vi "Named_Serial_Comms.vi"(0 "Channel Name":string, 1 "Write":string, 2 "Timeout/ms":u32=500, 4 "!Error retries":i32=10, 6 "!Timeout retries":i32=3, 9 "Port Name":refnum<visa-resource-name>, 11 "Term Grep":string="\r$", 12 "Log Errors?":bool=TRUE, 13 "Terminate Count":i32) -> (3 "Read":string="This is simulation mode", 8 "Error Description":string, 10 "millisecond timer value":u32, 14 "Timed out":bool, 15 "Serial Error":bool)   [LabVIEW 2022 SP3]
doc: "The Serial Communication VI performs bidirectional communication with a port. It initializes the port, writes a string to the port, and performs a read with timeout. The Read with Timeout will wait until a terminating character is received or the time limit is up, whichever comes first.\nThe initialisation parameters, terminating character, and timeout, are all set in the Serial Setup Global."
uses:
  subVIs/Port_Params.ctl
  <vilib>/Instr/_visa.llb/VISA Find Search Mode.ctl
  <vilib>/Instr/serial.llb/serpConfig.vi
  Anemometry/Anemometry Sub Vis/Globals/Preference_global.vi
panel:
  in  "Tab Control":T1(tab)
  in  "Uppercase?":bool
  in  "Append Return?":bool
  in  "!stop":bool
  out "Terminated?":bool
  in  "Force setup reload":bool
  in  "Save Setups?":bool
  out "Buffer Trash":string
  out "byte count":u32
  out "Port Settings Array":T2[](array[typedef]) {"flow control etc."."parity err byte" format="%.0x"; "flow control etc."."XON byte" format="%.0x"; "flow control etc."."XOFF byte" format="%.0x"; "data bits" min=5 max=8 step=1}
  out "enumerated ports":string[](array[string])
  out "Ports having file settings":string[](array[string])
  out "Port Initialised?":bool[](array[boolean])
  out "Setting Number":i32
  out "Port Initialisation Parameters":T2={"Name"="", "flow control etc."={"input XON/XOFF"=FALSE, "input HW Handshake"=FALSE, "input alt HW HShk"=FALSE, "output XON/XOFF"=FALSE, "output HW Handshake"=FALSE, "output alt HW HShk"=FALSE, "XOFF byte "=0, "XON byte"=0, "parity err byte"=0}, "buffer size"=0, "baud rate"=9600, "data bits"=8, "stop bits"=enum."1 bit", "parity"=enum."no parity"} {"flow control etc."."parity err byte" format="%.0x"; "flow control etc."."XON byte" format="%.0x"; "flow control etc."."XOFF byte" format="%.0x"; "data bits" min=5 max=8 step=1}
  out "isGillUsonic":bool
  out "etherComms":errorcluster
  out "Audit trail":string[](array[string])
  out "Case":string="Simulate"
  out "Initialise error":i32
  out "Write error":i32
  out "n-bytes error code":i32
  out "read error code":i32
  out "Close Port error":i32
  out "load setups error":bool
  out "PortType":string
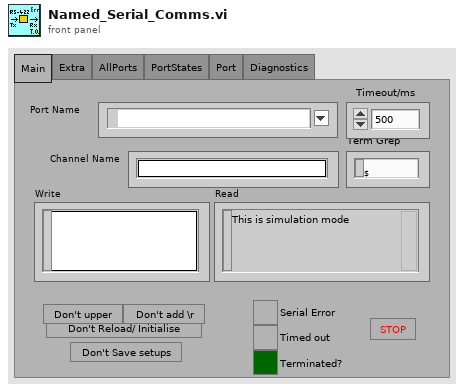
[diagram p1: front panel]
types:
  T1 = enum32{"Main", "Extra", "AllPorts", "PortStates", "Port", "Diagnostics"}
  T2 = typedef "Port_Params.ctl" = cluster{"Name":string, "flow control etc.":cluster{"input XON/XOFF":bool, "input HW Handshake":bool, "input alt HW HShk":bool, "output XON/XOFF":bool, "output HW Handshake":bool, "output alt HW HShk":bool, "XOFF byte ":u8, "XON byte":u8, "parity err byte":u16}, "buffer size":u16, "baud rate":u32, "data bits":u16, "stop bits":enum16{"1 bit", "1.5 bits", "2 bits"}, "parity":enum16{"no parity", "odd parity", "even parity", "mark parity", "space parity"}}
  T3 = typedef "VISA Find Search Mode.ctl" = u32
  T4 = cluster{"input XON/XOFF":bool, "input HW Handshake":bool, "input alt HW HShk":bool, "output XON/XOFF":bool, "output HW Handshake":bool, "output alt HW HShk":bool, "XOFF byte ":u8, "XON byte":u8, "parity err byte":u16}
  T5 = enum16{"no parity", "odd parity", "even parity", "mark parity", "space parity"}
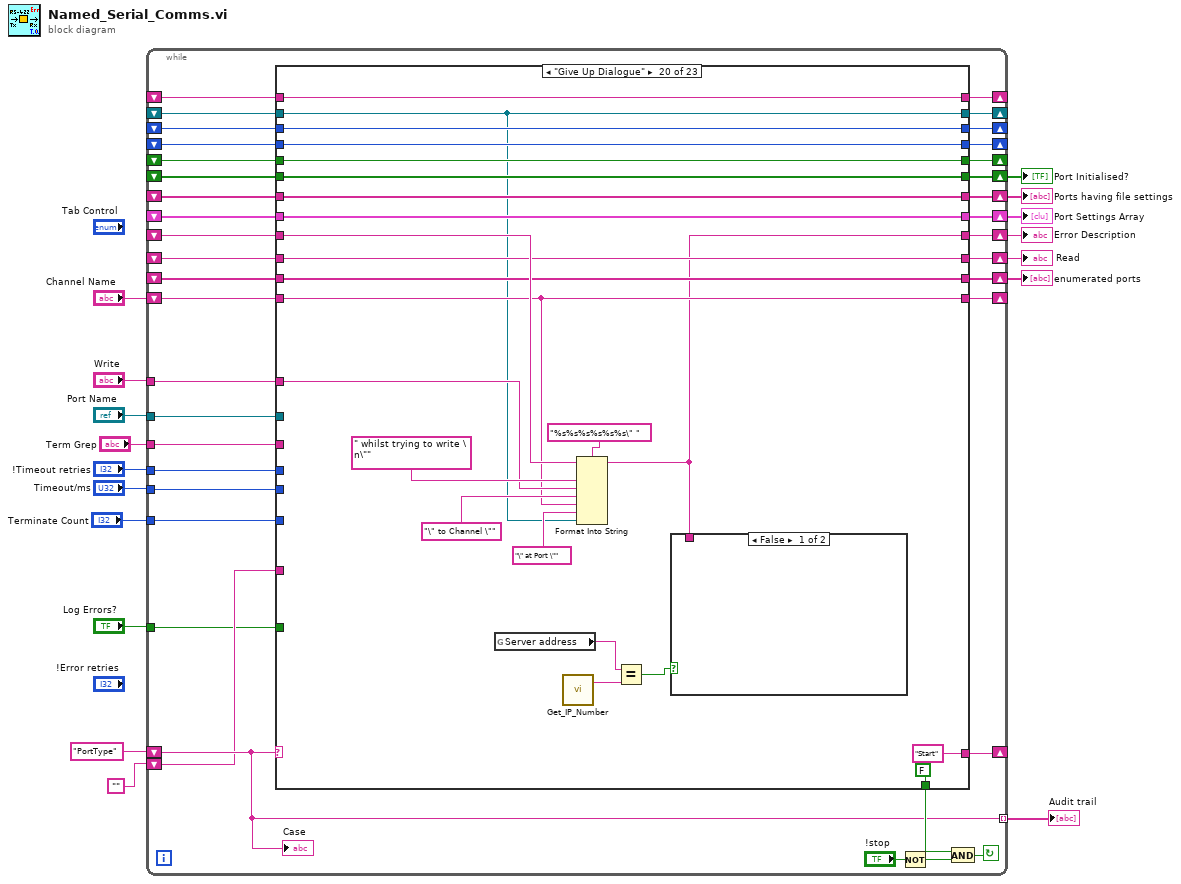
[diagram p0: block diagram]
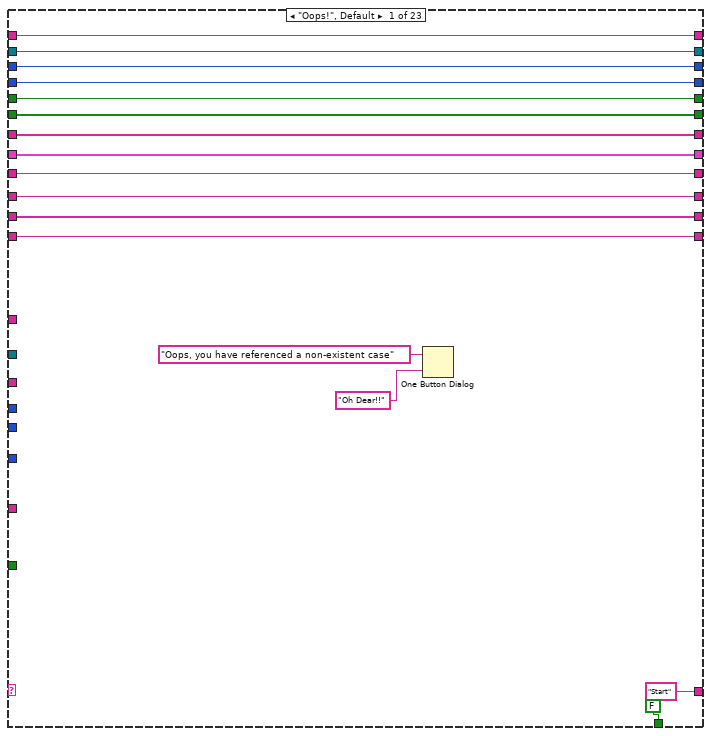
[diagram p2: hidden frame]
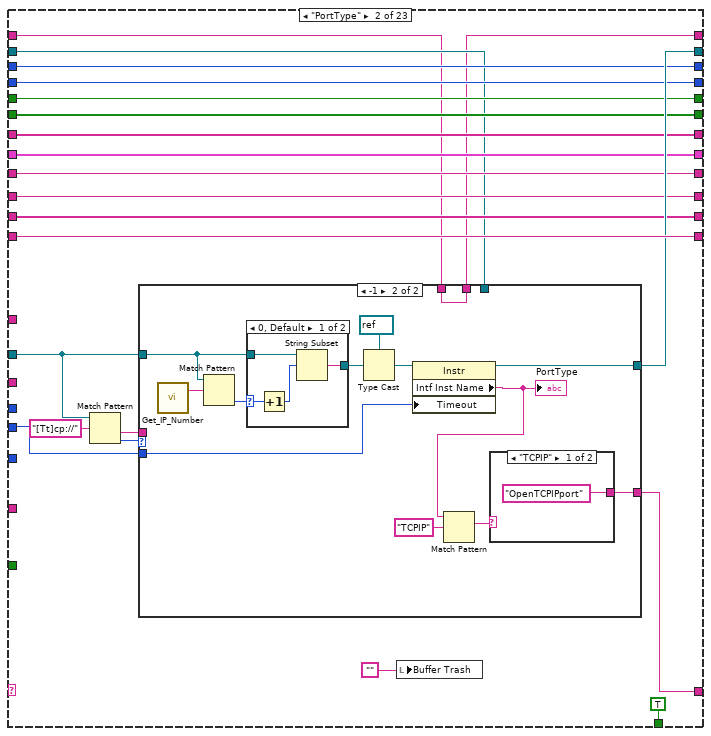
[diagram p3: hidden frame]
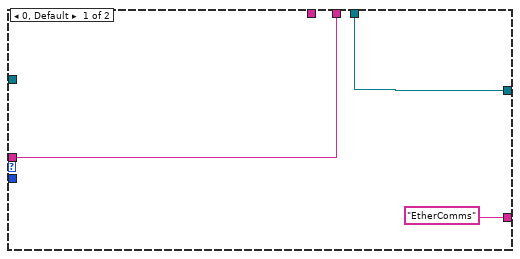
[diagram p4: hidden frame]
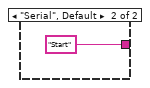
[diagram p5: hidden frame]
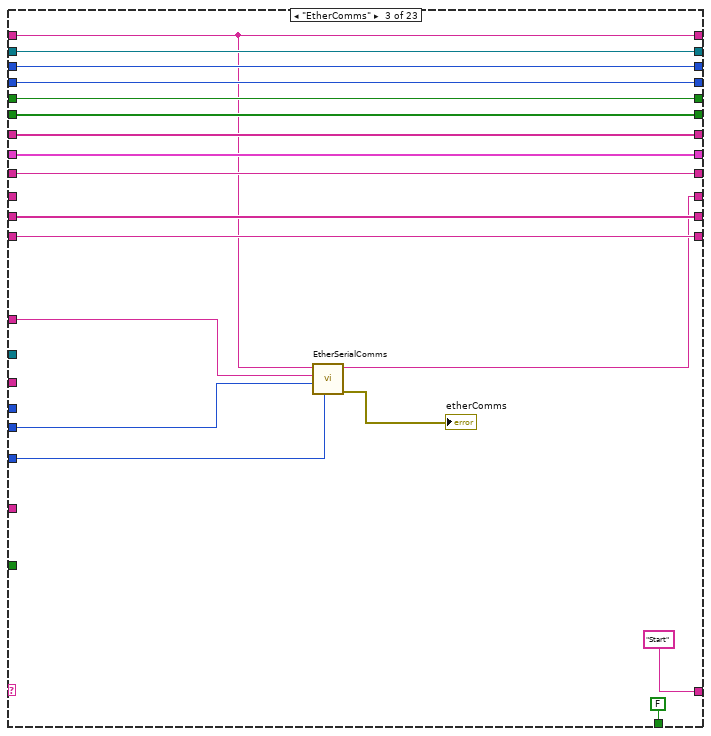
[diagram p7: hidden frame]
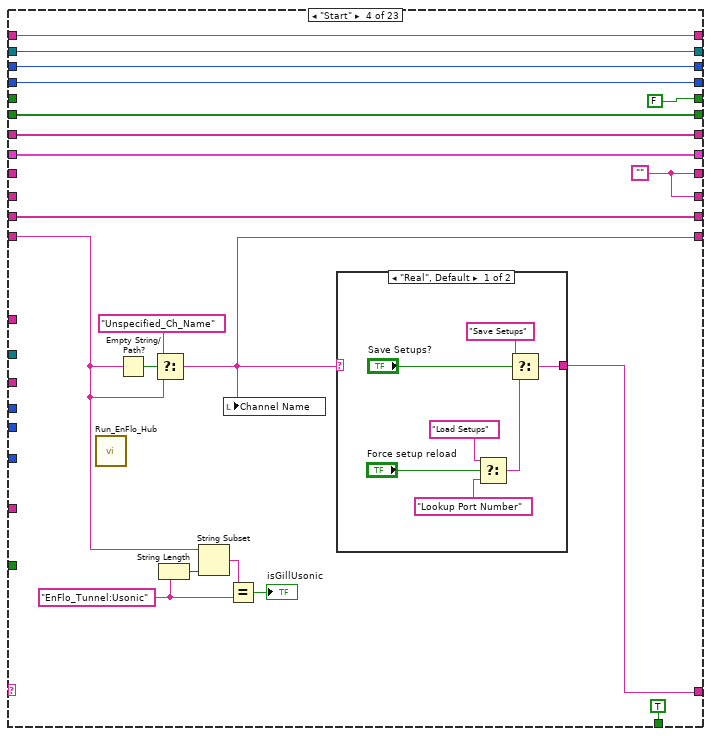
[diagram p8: hidden frame]
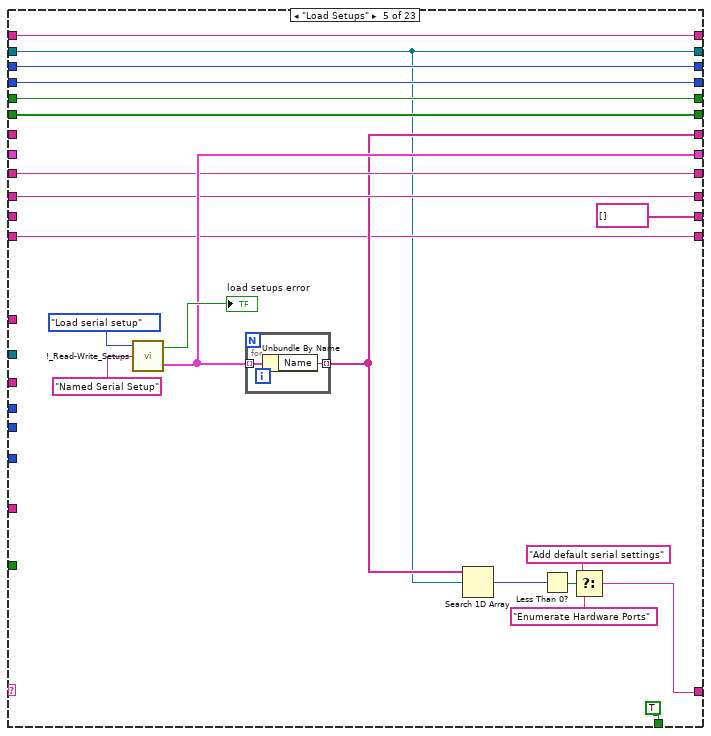
[diagram p10: hidden frame]
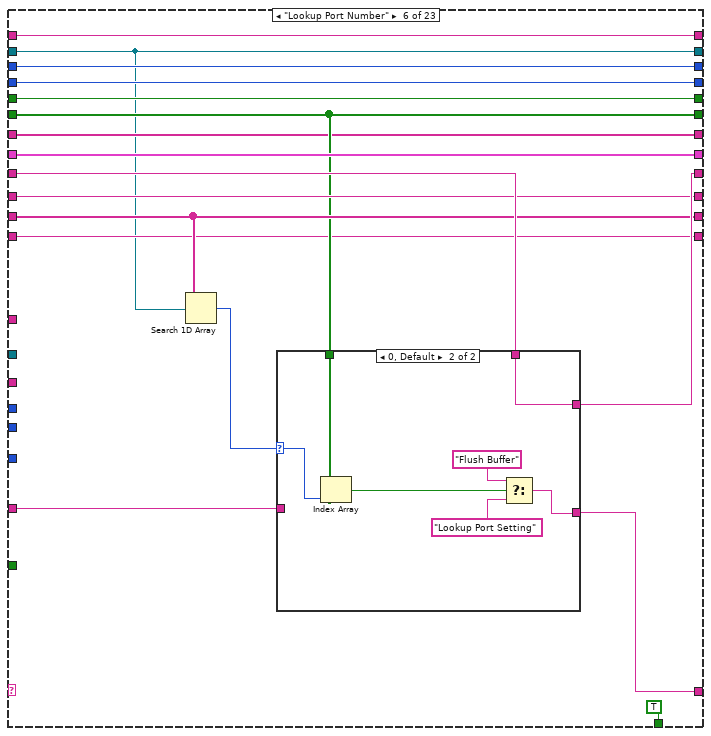
[diagram p11: hidden frame]
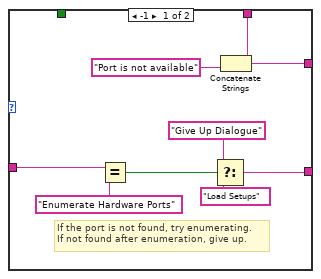
[diagram p12: hidden frame]
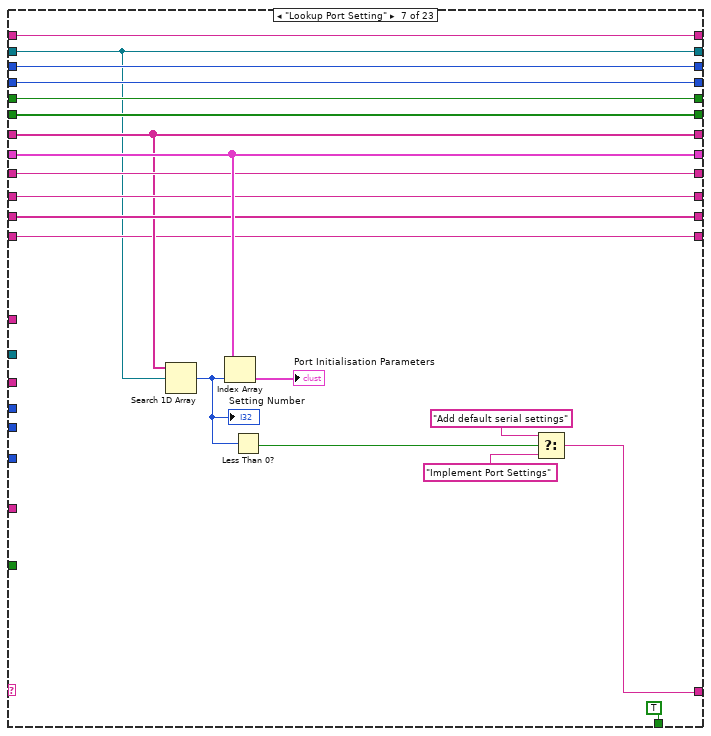
[diagram p13: hidden frame]
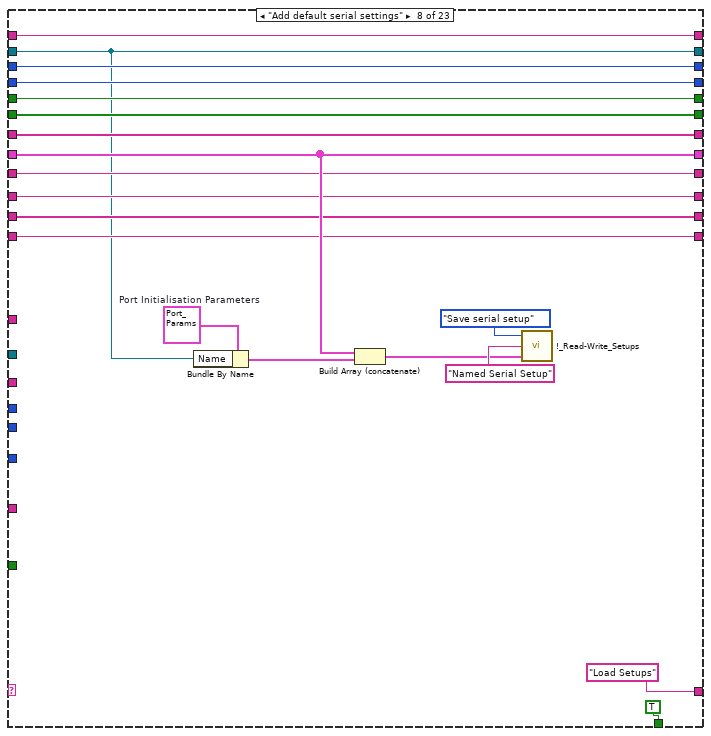
[diagram p14: hidden frame]
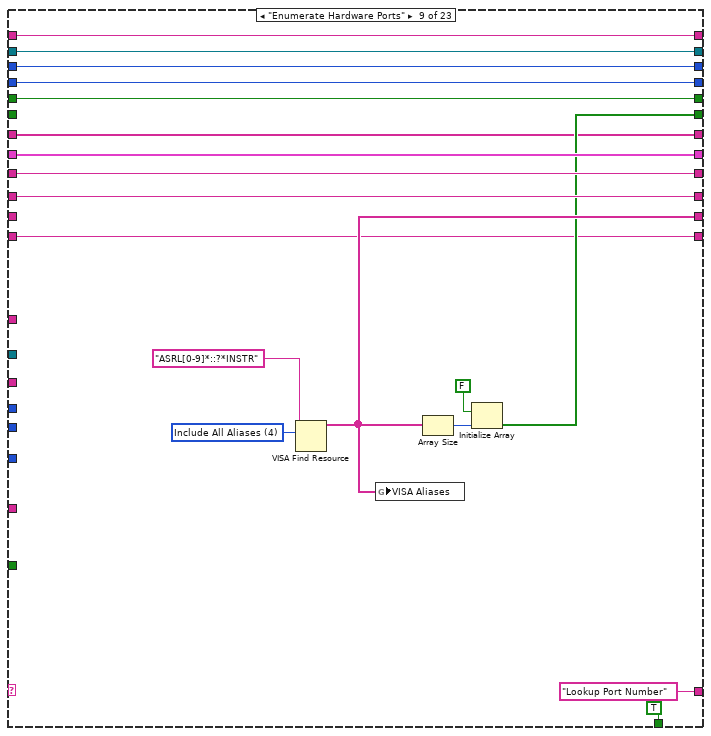
[diagram p15: hidden frame]
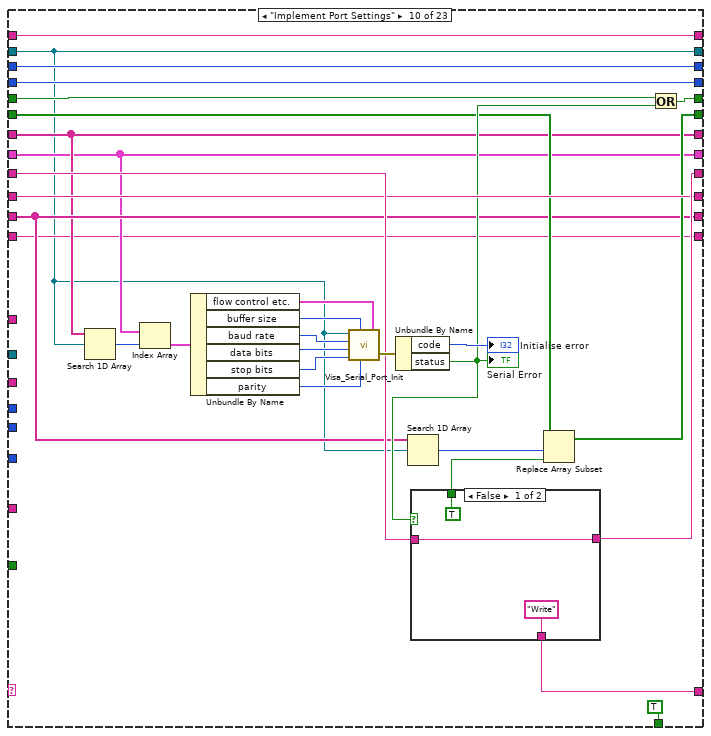
[diagram p16: hidden frame]
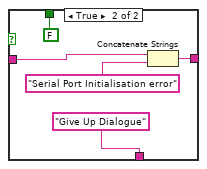
[diagram p17: hidden frame]
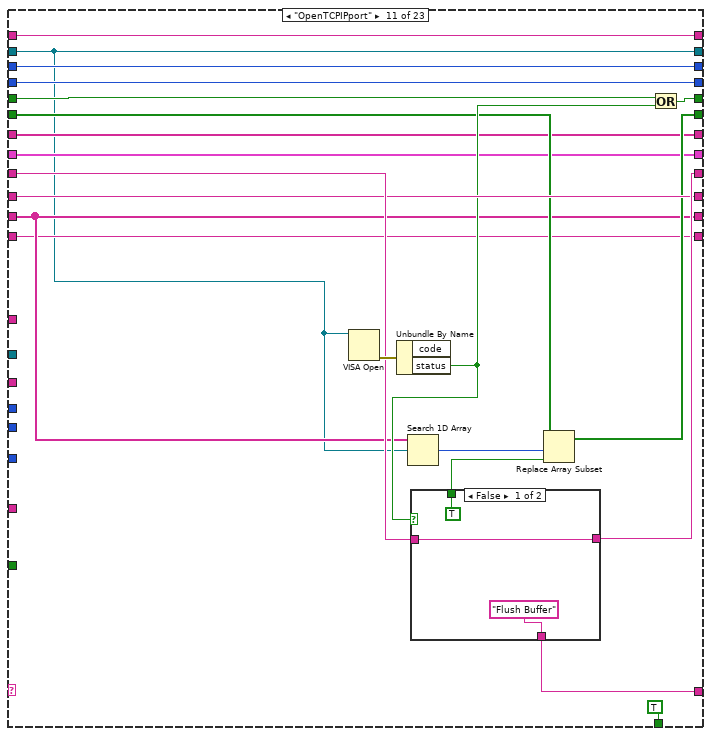
[diagram p18: hidden frame]
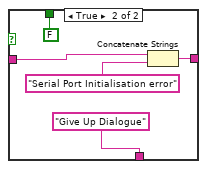
[diagram p19: hidden frame]
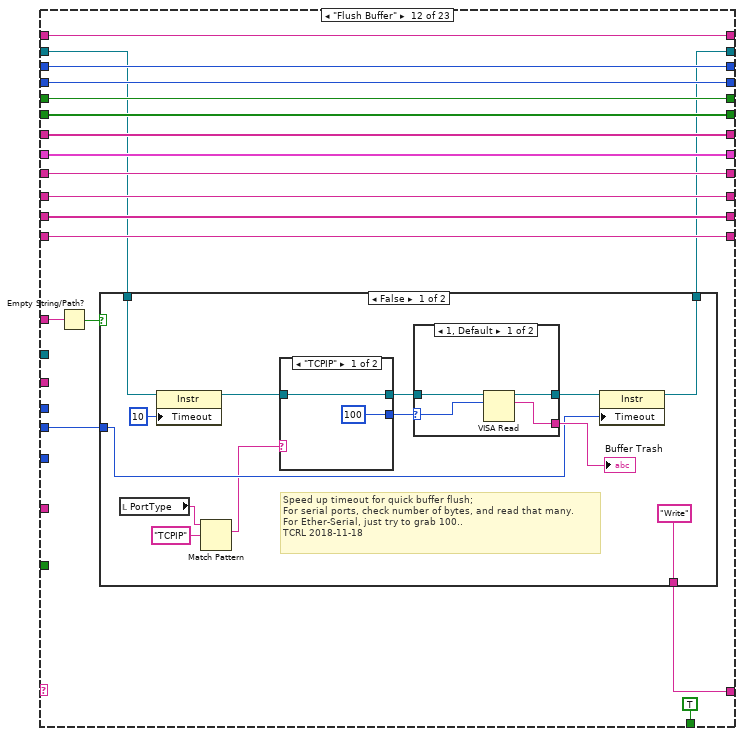
[diagram p20: hidden frame]
diagram:
  n1 = while {
    tunnel: "!Timeout retries" -> [w47]
    shift-left: "" -> [w48]
    tunnel: [w49] -> w5 mode=indexing
    shift-left: "PortType" -> [w49]
    shift-right: [w50] -> _
    tunnel: "Write" -> [w55]
    tunnel: "Log Errors?" -> [w46]
    shift-right: [w45] -> w12
    shift-left: _ -> [w44]
    shift-right: [w42] -> w11
    shift-left: _ -> [w43]
    shift-right: [w41] -> w10
    shift-left: _ -> [w40]
    shift-right: [w39] -> w9
    shift-left: _ -> [w38]
    shift-right: [w37] -> _
    shift-left: _ -> [w36]
    shift-right: [w35] -> w8
    shift-left: _ -> [w34]
    shift-right: [w32] -> w7
    shift-left: _ -> [w33]
    shift-right: [w29] -> _
    shift-left: _ -> [w28]
    shift-right: [w31] -> _
    shift-left: _ -> [w30]
    shift-right: [w26] -> _
    shift-left: "Channel Name" -> [w27]
    shift-right: [w25] -> _
    shift-left: _ -> [w24]
    tunnel: "Port Name" -> [w23]
    shift-right: [w22] -> _
    shift-left: _ -> [w21]
    tunnel: "Timeout/ms" -> [w20]
    tunnel: "Terminate Count" -> [w19]
    tunnel: "Term Grep" -> [w18]
    stop <- w53 continue-if-true
    n2 = case shown="\"Give Up Dialogue\"" w49 {
      tunnel: w55 -> [_ _ w121 _ _ _ _ _ _ _ _ w344 w405 _ _ _ _ _ w604 w631 _ _ _]
      tunnel: ["Start" ("f") w74 "Start" w154 w165 w201 w223 "Load Setups" ("f") "Lookup Port Number" w297 w332 w342 w402 "Bytes At Serial Port?" ("f") w472 w526 w552 w594 "Start" "Start" "Start" "Start" ("f") "Load Setups" ("f")] -> w50
      tunnel: [FALSE TRUE FALSE TRUE TRUE TRUE TRUE TRUE TRUE TRUE TRUE TRUE TRUE TRUE TRUE TRUE TRUE TRUE FALSE FALSE TRUE FALSE TRUE] -> w54
      tunnel: w48 -> [_ _ _ _ _ w200 _ _ _ _ _ _ _ _ _ _ _ _ _ _ _ _ _]
      tunnel: w47 -> [_ _ _ _ _ _ _ _ _ _ _ _ w400 _ w471 _ _ _ _ _ _ _ _]
      tunnel: w46 -> [_ _ _ _ _ _ _ _ _ _ _ _ _ _ _ _ _ _ w610 _ _ _ _]
      tunnel: [w67 w86 w128 w152 w179 w199 w234 w249 w270 w281 w318 w358 w399 w451 w470 w518 w547 w590 w609 w628 w650 w667 w681] -> w45
      tunnel: w44 -> [w67 w86 w128 w152 _ w199 w234 w249 w270 w281 w318 w358 w399 w451 w470 w518 w547 w590 w609 w628 w650 w667 w681]
      tunnel: w43 -> [w66 w85 w127 _ w178 w198 w233 w248 w269 w292 w328 w357 w397 w450 w469 w517 w546 w589 w608 w627 w649 w666 w680]
      tunnel: [w66 w85 w127 w151 w178 w197 w233 w248 w269 w293 w329 w357 w398 w450 w469 w517 w546 w589 w608 w616 w649 w666 w680] -> w42
      tunnel: [w65 w84 w119 w151 w177 w196 w232 w247 w268 w291 w327 w356 w396 "" w468 w516 w545 w588 w607 w626 w648 "Simulated Serial Read" w679] -> w41
      tunnel: w40 -> [w65 w84 _ _ w177 w196 w232 w247 w268 w291 w327 w356 w396 _ w468 w515 w545 w588 w607 w626 w648 _ w679]
      tunnel: [w64 w83 w126 w150 string[] [] ("enumerated ports") w195 w231 w246 w267 w283 w320 w355 w395 w448 w467 w514 w544 w587 w606 w625 w647 w664 w678] -> w39
      tunnel: w38 -> [w64 w83 w126 w150 _ w195 w231 w246 _ w283 w320 w355 w395 w448 w467 w514 w544 w587 w606 w625 w647 w664 w678]
      tunnel: [w63 w89 w131 FALSE w175 w194 w230 w245 w266 w289 w325 w354 w394 w447 w466 w513 w543 w585 w605 w624 w646 w663 w677] -> w37
      tunnel: w36 -> [w63 w89 w131 _ w175 w194 w230 w245 w266 w290 w326 w354 w394 w447 w466 w513 w543 w586 w605 w624 w646 w663 w677]
      tunnel: [w62 w88 w130 w148 w174 w192 w229 w244 w265 w286 w322 w353 w393 w446 w465 w512 w542 w583 w603 w623 w645 w662 w676] -> w35
      tunnel: w34 -> [w62 w88 w130 w148 w174 w192 w229 w244 _ w285 w321 w353 w393 w446 w465 w512 w542 w583 w603 w623 w645 w662 w676]
      tunnel: [w61 w87 w129 w147 w173 w191 w228 w243 w264 w282 w319 w352 w392 w445 w464 w511 w541 w582 w602 w622 w644 w661 w675] -> w32
      tunnel: w33 -> [w61 w87 w129 w147 _ w191 w228 w243 w264 w282 w319 w352 w392 w445 w464 w511 w541 w582 w602 w622 w644 w661 w675]
      tunnel: [w60 w91 w133 w146 w172 w190 w227 w242 w263 w279 w317 w351 w391 w444 w462 w507 w540 w581 w601 w621 w643 w660 w674] -> w31
      tunnel: w30 -> [w60 w91 w133 w146 w172 w190 w227 w242 w263 w279 w317 w351 w391 _ w462 w507 w540 w581 w601 w621 w643 w660 w674]
      tunnel: [w59 w90 w132 w145 w171 w189 w226 w241 w262 w278 w316 w350 w390 w443 w463 w506 w539 w580 w600 w620 w642 w659 w673] -> w29
      tunnel: w28 -> [w59 w90 w132 w145 w171 w189 w226 w241 w262 w278 w316 w350 w390 w443 _ w506 w539 w580 w600 w620 w642 w659 w673]
      tunnel: w27 -> [w58 w93 w134 w137 w170 w188 w225 w240 w260 w277 w315 w349 w388 w442 w461 w505 w538 w579 w597 w619 w641 w658 w672]
      tunnel: [w58 w93 w134 w135 w170 w188 w225 w240 w260 w277 w315 w349 w388 w442 w461 w505 w538 w579 w597 w619 w641 w658 w672] -> w26
      tunnel: [w57 w92 w123 w142 w164 w187 w221 w239 w259 w276 w313 w346 w387 w441 w459 w504 w537 w578 w599 w618 w640 w657 w671] -> w25
      tunnel: w24 -> [w57 w77 w123 w142 w164 w187 w221 w239 w259 w276 w313 w345 w387 w441 w459 w504 w537 w578 w599 w618 w640 w657 w671]
      tunnel: w23 -> [_ w81 _ _ _ _ _ _ _ _ _ _ _ _ _ _ _ _ _ _ _ _ _]
      tunnel: [w56 w76 w122 w141 w163 w186 w222 w238 w258 w275 w314 w348 w386 w440 w460 w503 w536 w577 w598 w617 w639 w656 w670] -> w22
      tunnel: w21 -> [w56 w75 w122 w141 w163 w186 w222 w238 w258 w275 w314 w348 w386 w440 w460 w503 w536 w577 w598 w617 w639 w656 w670]
      tunnel: w20 -> [_ w73 w120 _ _ _ _ _ _ _ _ w347 _ _ _ _ _ w576 _ _ _ _ _]
      tunnel: w19 -> [_ _ w117 _ _ _ _ _ _ _ _ _ _ _ w458 _ w535 _ _ _ _ _ _]
      tunnel: w18 -> [_ _ _ _ _ _ _ _ _ _ _ _ _ _ w457 _ w534 _ _ _ _ _ _]
      frame "Oops!", Default {
        n3 = One Button Dialog(message="Oops, you have referenced a non-existent case", button name ("OK")="Oh Dear!!") -> ()  [unwired: 1 out]
      }
      frame "PortType" {
        n4 = Match Pattern(string=w81, regular expression="[Tt]cp://") -> (after substring=w78:string, offset past match=w79:i32)  [unwired: 1 in, 2 out]
        n5 = case shown="-1" w79 {
          tunnel: [w96 w100] -> w92
          tunnel: w81 -> [_ w105]
          tunnel: w78 -> [w95 _]
          tunnel: w77 -> [w96 _]
          tunnel: [w95 w104] -> w76
          tunnel: w75 -> [_ w104]
          tunnel: ["EtherComms" w103] -> w74
          tunnel: w73 -> [_ w102]
          frame 0, Default {
          }
          frame -1 {
            n6 = call "Get_IP_Number.vi"() -> ("IP Number"=w108:string)  [unwired: 1 out]
            n7 = Match Pattern(string=w105, regular expression=w108) -> (offset past match=w107:i32)  [unwired: 4 out]
            n8 = case shown="0, Default" w107 {
              selector: w107 -> [w112 _]
              tunnel: [w113 w116] -> w109
              tunnel: w105 -> [w114 w116]
              frame 0, Default {
                n9 = Increment(x=w112) -> (x+1=w115:i32)
                n10 = String Subset(string=w114, offset (0)=w115) -> (substring=w113:string)  [unwired: 1 out]
              }
              frame -1 {
              }
            }
            n11 = Type Cast(type=refnum<visa-resource-name> refnum ("dup VISA resource name"), x=w109) -> (*(type *) &x=w101:refnum<visa-resource-name>)
            n12 = property class="Instr"(reference=w101, "Timeout"=w102) -> (reference out=w100:refnum<visa-resource-name>, "Intf Inst Name"=w97:string)  [unwired: 1 in, 1 out]
            "PortType" <- w97
            n13 = Match Pattern(string=w97, regular expression="TCPIP") -> (match substring=w98:string)  [unwired: 1 in, 3 out]
            n14 = case shown="\"TCPIP\"" w98 {
              tunnel: ["OpenTCPIPport" "Start"] -> w103
              frame "TCPIP" {
              }
              frame "Serial", Default {
              }
            }
          }
        }
        n15 = local write "Buffer Trash"("") -> ()
      }
      frame "EtherComms" {
        n16 = call "EtherSerialComms.vi"("byteCount"=w117, "Timeout/ms"=w120, "Write"=w121, "Port Name"=w122) -> ("error out"=→"etherComms":errorcluster, "data out"=w119:string)  [unwired: 5 in, 1 out]
      }
      frame "Start" {
        w140 = "EnFlo_Tunnel:Usonic"
        w151 = ""
        n17 = call "Run_EnFlo_Hub.vi"() -> ()  [unwired: 1 in, 7 out]
        n18 = Empty String/Path?(string/path=w137) -> (empty?=w144:bool)
        n19 = Select(t="Unspecified_Ch_Name", s=w144, f=w137) -> (s? t:f=w135:string)
        n20 = String Length(string=w140) -> (length=w138:i32)
        n21 = String Subset(string=w137, length (rest)=w138) -> (substring=w139:string)  [unwired: 1 out]
        n22 = local write "Channel Name"(w135) -> ()
        n23 = Equal?(x=w139, y=w140) -> (x = y?=→"isGillUsonic":bool)
        n24 = case shown="\"Real\", Default" w135 {
          selector: w135 -> [_ w162]
          tunnel: [w157 w162] -> w154
          frame "Real", Default {
            n25 = Select(t="Load Setups" ("f"), s="Force setup reload", f="Lookup Port Number") -> (s? t:f=w158:string)
            n26 = Select(t="Save Setups", s="Save Setups?", f=w158) -> (s? t:f=w157:string)
          }
          frame "Simulate" {
          }
        }
      }
      frame "Load Setups" {
        n27 = call "!_Read-Write_Setups.vi"("Setup Name"="Named Serial Setup", "Mode"=enum16{"Load serial setup", "Save serial setup"}."Load serial setup") -> ("Port Settings Array Out"=w179:T2[], "error unflattening"=→"load setups error":bool)  [unwired: 1 in]
        n28 = for {
          tunnel: w179 -> [w185] mode=indexing
          tunnel: [w184] -> w173 mode=indexing
          n29 = Unbundle By Name(w185) -> ("Name"=w184:string)
        }
        n30 = Search 1D Array(1D array=w173, element=w164) -> (index of element=w169:i32)  [unwired: 1 out]
        n31 = Less Than 0?(x=w169) -> (x < 0?=w168:bool)
        n32 = Select(t="Add default serial settings", s=w168, f="Enumerate Hardware Ports") -> (s? t:f=w165:string)
      }
      frame "Lookup Port Number" {
        n33 = Search 1D Array(1D array=w195, element=w187) -> (index of element=w193:i32)  [unwired: 1 out]
        n34 = case shown="0, Default" w193 {
          selector: w193 -> [_ w212]
          tunnel: [w211 w218] -> w201
          tunnel: w200 -> [w208 _]
          tunnel: w198 -> [w204 w214]
          tunnel: [w203 w214] -> w197
          tunnel: w192 -> [_ w213]
          frame -1 {
            # "If the port is not found, try enumerating.\nIf not found after enumeration, give up."
            n35 = Equal?(x=w208, y="Enumerate Hardware Ports" ("f")) -> (x = y?=w210:bool)
            n36 = Select(t="Give Up Dialogue" ("f"), s=w210, f="Load Setups") -> (s? t:f=w211:string)
            n37 = Concatenate Strings(w204, "Port is not available" ("Error Description")) -> (w203:string)
          }
          frame 0, Default {
            n38 = Index Array(array=w213, index=w212) -> (element=w217:bool)
            n39 = Select(t="Flush Buffer" ("f"), s=w217, f="Lookup Port Setting") -> (s? t:f=w218:string)
          }
        }
      }
      frame "Lookup Port Setting" {
        n40 = Search 1D Array(1D array=w228, element=w221) -> (index of element=w235:i32)  [unwired: 1 out]
        "Setting Number" <- w235
        n41 = Index Array(array=w234, index=w235) -> (element=→"Port Initialisation Parameters":T2)
        n42 = Less Than 0?(x=w235) -> (x < 0?=w224:bool)
        n43 = Select(t="Add default serial settings", s=w224, f="Implement Port Settings") -> (s? t:f=w223:string)
      }
      frame "Add default serial settings" {
        w256 = T2 {"Name"="", "flow control etc."={"input XON/XOFF"=FALSE, "input HW Handshake"=FALSE, "input alt HW HShk"=FALSE, "output XON/XOFF"=FALSE, "output HW Handshake"=FALSE, "output alt HW HShk"=FALSE, "XOFF byte "=19, "XON byte"=17, "parity err byte"=0}, "buffer size"=200, "baud rate"=9600, "data bits"=8, "stop bits"=enum."1 bit", "parity"=enum."no parity"}  # Port Initialisation Parameters
        n44 = Bundle By Name(cluster=w256, "Name"=w239) -> (w255:T2)
        n45 = Build Array (concatenate)(w249, w255) -> (w252:T2[])
        n46 = call "!_Read-Write_Setups.vi"("Port Settings Array In"=w252, "Setup Name"="Named Serial Setup", "Mode"=enum16{"Load serial setup", "Save serial setup"}."Save serial setup") -> ()  [unwired: 2 out]
      }
      frame "Enumerate Hardware Ports" {
        w261 = T3 4 items=["Canonical Names Only"=0, "Aliases Only"=2, "Include Matching Aliases"=3, "Include All Aliases"=4] ("Search Mode")
        n47 = VISA Find Resource(10:w261, 11:"ASRL[0-9]*::?*INSTR" ("expression (\"?*\")")) -> (3:w267:string[])  [unwired: 1 in, 2 out]
        n48 = global write "serpConfig.vi" "VISA Aliases"(w267) -> ()
        n49 = Array Size(array=w267) -> (size(s)=w272:i32)
        n50 = Initialize Array(FALSE, w272) -> (w265:bool[])
      }
      frame "Implement Port Settings" {
        n51 = Search 1D Array(1D array=w282, element=w276) -> (index of element=w284:i32)  [unwired: 1 out]
        n52 = Index Array(array=w281, index=w284) -> (element=w280:T2)
        n53 = Unbundle By Name(w280) -> ("flow control etc."=w304:T4, "buffer size"=w303:u16, "baud rate"=w302:u32, "data bits"=w301:u16, "stop bits"=w300:enum16{"1 bit", "1.5 bits", "2 bits"}, "parity"=w299:T5)
        n54 = call "Visa_Serial_Port_Init.vi"("flow control etc."=w304, "parity"=w299, "buffer size"=w303, "stop bits"=w300, "data bits"=w301, "baud rate"=w302, "Visa Port Name"=w276) -> ("error out"=w295:errorcluster)
        n55 = Unbundle By Name(w295) -> ("code"=→"Initialise error":i32, "status"=w288:bool)
        "Serial Error" <- w288
        n56 = Search 1D Array(1D array=w283, element=w276) -> (index of element=w287:i32)  [unwired: 1 out]
        n57 = case shown="False" w288 {
          tunnel: ["Write" "Give Up Dialogue"] -> w297
          tunnel: [TRUE ("Element Data") FALSE ("Element Data")] -> w296
          tunnel: [w305 w309] -> w293
          tunnel: w292 -> [w305 w308]
          frame False {
          }
          frame True {
            n58 = Concatenate Strings(w308, "Serial Port Initialisation error" ("Error Description")) -> (w309:string)
          }
        }
        n59 = Replace Array Subset(array=w285, new element=w296, index=w287) -> (w286:bool[])
        n60 = Or(x=w290, y=w288) -> (x .or. y?=w289:bool)
      }
      frame "OpenTCPIPport" {
        n61 = VISA Open(VISA resource name=w313) -> (error out=w330:errorcluster)  [unwired: 4 in, 1 out]
        n62 = Unbundle By Name(w330) -> ("status"=w324:bool)  [unwired: 1 out]
        n63 = Search 1D Array(1D array=w320, element=w313) -> (index of element=w323:i32)  [unwired: 1 out]
        n64 = case shown="False" w324 {
          tunnel: ["Flush Buffer" "Give Up Dialogue"] -> w332
          tunnel: [TRUE ("Element Data") FALSE ("Element Data")] -> w331
          tunnel: [w334 w338] -> w329
          tunnel: w328 -> [w334 w337]
          frame False {
          }
          frame True {
            n65 = Concatenate Strings(w337, "Serial Port Initialisation error" ("Error Description")) -> (w338:string)
          }
        }
        n66 = Replace Array Subset(array=w321, new element=w331, index=w323) -> (w322:bool[])
        n67 = Or(x=w326, y=w324) -> (x .or. y?=w325:bool)
      }
      frame "Flush Buffer" {
        n68 = Empty String/Path?(string/path=w344) -> (empty?=w343:bool)
        n69 = case shown="False" w343 {
          tunnel: w347 -> [w366 _]
          tunnel: [w365 w385] -> w346
          tunnel: w345 -> [w364 w385]
          tunnel: ["Write" ("f") "Start Read loop" ("f")] -> w342
          frame False {
            # "Speed up timeout for quick buffer flush;\nFor serial ports, check number of bytes, and read that many.\nFor Ether-Serial, just try to grab 100..\nTCRL 2018-11-18"
            n70 = local read "PortType"() -> (w362:string)
            n71 = property class="Instr"(reference=w364, "Timeout"=u32 10 ("General Settings:Timeout Value")) -> (reference out=w370:refnum<visa-resource-name>)  [unwired: 1 in, 1 out]
            n72 = Match Pattern(string=w362, regular expression="TCPIP") -> (match substring=w360:string)  [unwired: 1 in, 3 out]
            n73 = case shown="\"TCPIP\"" w360 {
              tunnel: [u32 100 ("Bytes at Port") w377] -> w371
              tunnel: w370 -> [w374 w376]
              tunnel: [w374 w375] -> w369
              frame "TCPIP" {
              }
              frame "Serial", Default {
                n74 = property class="Instr"(reference=w376) -> (reference out=w375:refnum<visa-resource-name>, "Serial Settings:Number of Bytes at Serial Port"=w377:u32)  [unwired: 1 in, 1 out]
              }
            }
            n75 = case shown="1, Default" w371 {
              selector: w371 -> [w379 _]
              tunnel: [w381 ""] -> w372
              tunnel: w369 -> [w380 w382]
              tunnel: [w378 w382] -> w367
              frame 1, Default {
                n76 = VISA Read(VISA resource name=w380, byte count=w379) -> (VISA resource name out=w378:refnum<visa-resource-name>, read buffer=w381:string)  [unwired: 1 in, 2 out]
              }
              frame 0 {
              }
            }
            "Buffer Trash" <- w372
            n77 = property class="Instr"(reference=w367, "Timeout"=w366) -> (reference out=w365:refnum<visa-resource-name>)  [unwired: 1 in, 1 out]
          }
          frame True {
            # "Don't flush buffer for an empty write, as this is an instrument which pushes data without being polled. We'll take what's in the buffer...\n\nTCRL 2018-11-18"
          }
        }
      }
      frame "Write" {
        n78 = case shown="False" "Uppercase?" {
          tunnel: w405 -> [w437 w439]
          tunnel: [w437 w438] -> w407
          frame False {
          }
          frame True {
            n79 = To Upper Case(1:w439) -> (0:w438:string)
          }
        }
        n80 = case shown="False" "Append Return?" {
          tunnel: w407 -> [w433 w436]
          tunnel: [w433 w435] -> w404
          frame False {
          }
          frame True {
            n81 = Concatenate Strings(w436, "\r") -> (w435:string)
          }
        }
        n82 = while {
          tunnel: w400 -> [w418]
          tunnel: [w409] -> w401
          tunnel: w404 -> [w416]
          tunnel: w387 -> [w415]
          tunnel: [w414] -> w389
          i -> [w422]
          stop <- w419 continue-if-true
          n83 = VISA Write(VISA resource name=w415, write buffer=w416) -> (error out=w417:errorcluster)  [unwired: 1 in, 2 out]
          n84 = Less?(x=w422, y=w418) -> (x < y?=w421:bool)
          n85 = Unbundle By Name(w417) -> ("code"=w411:i32)
          n86 = Not Equal?(x=w411, y=-1073807298 ("code")) -> (x != y?=w412:bool)
          n87 = Tick Count (ms)() -> (millisecond timer value=w414:u32)
          n88 = Select(t=w411, s=w412, f=0) -> (s? t:f=w409:i32)
          n89 = Not Equal To 0?(x=w409) -> (x != 0?=w420:bool)
          n90 = Compound Arithmetic op=AND(w420, w421) -> (w419:bool)
        }
        "Write error" <- w401
        "millisecond timer value" <- w389
        n91 = case shown="0" w401 {
          tunnel: ["Start Read loop" "Give Up Dialogue" "Give Up Dialogue"] -> w402
          tunnel: [w423 w426 w429] -> w398
          tunnel: w397 -> [w423 w425 w431]
          frame 0 {
            # "No error"
          }
          frame 5000, Default {
            # "Unspecified error; use code 5000 as this is the first user defined error code"
            n92 = Concatenate Strings(w425, "Unspecified Serial error at Write" ("Error Description")) -> (w426:string)
          }
          frame 37 {
            # "Port not found"
            n93 = Concatenate Strings(w431, "Port not found at Write" ("Error Description")) -> (w429:string)
          }
        }
      }
      frame "Start Read loop" {
        n94 = Tick Count (ms)() -> (millisecond timer value=w444:u32)
      }
      frame "Bytes At Serial Port?" {
        n95 = local read "PortType"() -> (w455:string)
        n96 = Match Pattern(string=w455, regular expression="TCPIP") -> (match substring=w454:string)  [unwired: 1 in, 3 out]
        n97 = case shown="\"Serial\", Default" w454 {
          tunnel: [TRUE w488] -> w475
          tunnel: ["Serial Port Read" ("f") w487] -> w473
          tunnel: w471 -> [_ w486]
          tunnel: [w477 w485] -> w463
          tunnel: w459 -> [_ w484]
          tunnel: w458 -> [w478 _]
          tunnel: w457 -> [w479 _]
          frame "TCPIP" {
            # "TCP VISA ports don't allow checking of BytesAtSerialPort. Therefore, if waiting for a terminator on a messgae of unknown length, read single bytes at a time, to avoid timing out trying to read too many.\nIf message is unterminated/ fixed-length, read fixed number of bytes.\nTCRL 2018-11-18"
            n98 = Empty String/Path?(string/path=w479) -> (empty?=w481:bool)
            n99 = Select(t=w478, s=w481, f=u32 1 ("Bytes at Port")) -> (s? t:f=w477:u32)
          }
          frame "Serial", Default {
            # "#Yuk Shouldn't use \"Timeout retries\" to say how many times to check for bytes at port!"
            n100 = while {
              tunnel: w486 -> [w493]
              tunnel: [w490] -> w485
              tunnel: [w494] -> w488
              tunnel: w484 -> [w491]
              i -> [w497]
              stop <- w495 continue-if-true
              n101 = property class="Instr"(reference=w491) -> (error out=w489:errorcluster, "Serial Settings:Number of Bytes at Serial Port"=w490:u32)  [unwired: 1 in, 1 out]
              "byte count" <- w490
              n102 = Unbundle By Name(w489) -> ("code"=w492:i32)
              "n-bytes error code" <- w492
              n103 = Less?(x=w497, y=w493) -> (x < y?=w496:bool)
              n104 = Equal To 0?(x=w492) -> (x = 0?=w494:bool)
              n105 = Compound Arithmetic op=AND(invert w494, w496) -> (w495:bool)
              n106 = case shown="True" w495 {
                frame False {
                }
                frame True {
                  n107 = Wait (ms)(milliseconds to wait=u32 5) -> ()  [unwired: 1 out]
                }
              }
            }
            n108 = case shown="0" w485 {
              tunnel: ["Serial Port Read" ("f") "Check for Termination" ("f")] -> w487
              frame 1, Default {
              }
              frame 0 {
                n109 = Wait (ms)(milliseconds to wait=u32 1) -> ()  [unwired: 1 out]
              }
            }
          }
        }
        n110 = Select(t=w473, s=w475, f="Log") -> (s? t:f=w472:string)
      }
      frame "Serial Port Read" {
        n111 = local read "isGillUsonic"() -> (w502:bool)
        n112 = Greater?(x=w506, y=u32 1) -> (0:w522:bool)
        n113 = And(x=w522, y=w502) -> (x .and. y?=w521:bool)
        n114 = case shown="True" w521 {
          tunnel: w506 -> [w531 w533]
          tunnel: [w531 w532] -> w508
          frame False {
          }
          frame True {
            n115 = Decrement(x=w533) -> (x-1=w532:u32)
          }
        }
        n116 = VISA Read(VISA resource name=w504, byte count=w508) -> (read buffer=w509:string, error out=w510:errorcluster)  [unwired: 1 in, 2 out]
        n117 = Unbundle By Name(w510) -> ("code"=w520:i32)
        n118 = case shown="1073676294" w520 {
          selector: w520 -> [w529 _]
          tunnel: [w529 0 ("code")] -> w519
          frame 0, Default {
          }
          frame 1073676294 {
          }
        }
        "read error code" <- w519
        n119 = Concatenate Strings(w515, w509) -> (w516:string)
        n120 = Equal To 0?(x=w519) -> (x = 0?=w525:bool)
        n121 = Select(t="Check for Termination" ("f"), s=w525, f="Log") -> (s? t:f=w526:string)
      }
      frame "Check for Termination" {
        n122 = Empty String/Path?(string/path=w534) -> (empty?=w554:bool)
        n123 = case shown="False" w554 {
          tunnel: w535 -> [w558 w573]
          tunnel: w545 -> [w560 w574]
          tunnel: [w555 w572] -> w551
          tunnel: w534 -> [w561 _]
          frame False {
            n124 = Decrement(x=w558) -> (x-1=w557:i32)
            n125 = while {
              tunnel: [w562] -> w556
              tunnel: w557 -> [w565]
              shift-left: 0 -> [w569]
              shift-right: [w568] -> _
              tunnel: w560 -> [w570]
              tunnel: w561 -> [w571]
              i -> [w566]
              stop <- w563 continue-if-true
              n126 = Match Pattern(string=w570, regular expression=w571, offset (0)=w569) -> (match substring=w562:string, offset past match=w568:i32)  [unwired: 2 out]
              n127 = Less?(x=w566, y=w565) -> (x < y?=w564:bool)
              n128 = Greater Or Equal To 0?(x=w568) -> (x >= 0?=w567:bool)
              n129 = Compound Arithmetic op=AND(w567, w564) -> (w563:bool)
            }
            n130 = Empty String/Path?(string/path=w556) -> (empty?=w555:bool)
          }
          frame True {
            n131 = String Length(string=w574) -> (length=w575:i32)
            n132 = Less?(x=w575, y=w573) -> (x < y?=w572:bool)
          }
        }
        n133 = Not(x=w551) -> (.not. x?=w548:bool)
        "Terminated?" <- w548
        n134 = Select(t="Log" ("f"), s=w548, f="TimeOut?") -> (s? t:f=w552:string)
      }
      frame "TimeOut?" {
        n135 = Tick Count (ms)() -> (millisecond timer value=w595:u32)
        n136 = Subtract(x=w595, y=w581) -> (x-y=w596:u32)
        n137 = Greater?(x=w596, y=w576) -> (0:w584:bool)
        "Timed out" <- w584
        n138 = Select(t="Log" ("f"), s=w584, f="Bytes At Serial Port?") -> (s? t:f=w594:string)
        n139 = Or(x=w586, y=w584) -> (x .or. y?=w585:bool)
      }
      frame "Log" {
        n140 = call "!_Serial_log_builder.vi"("Port Name"=w599, "Comms Error"=w605, "Channel Name"=w597, "Write String"=w604, "Log Errors?"=w610, "Read"=w607) -> ()  [unwired: 3 out]
      }
      frame "Give Up Dialogue" {
        n141 = global read "Preference_global.vi" "Server address"() -> (w614:string)
        n142 = call "Get_IP_Number.vi"() -> ("IP Number"=w615:string)  [unwired: 1 out]
        n143 = Format Into String(format string="%s%s%s%s%s%s\" ", initial string=w627, " whilst trying to write \n\"", w631, "\" to Channel \"", w619, "\" at Port \"" ("Input 5"), w618) -> (resulting string=w616:string)  [unwired: 1 in, 1 out]
        n144 = Equal?(x=w614, y=w615) -> (x = y?=w613:bool)
        n145 = case shown="False" w613 {
          tunnel: w616 -> [_ w636]
          frame False {
          }
          frame True {
            n146 = call "Server_Emails.vi"("Message"=w636, "Contact All clients?"=TRUE, "Subject"="Serial_Comms_Error") -> ()  [unwired: 2 in, 3 out]
          }
        }
      }
      frame "Close All Ports" {
        n147 = for {
          tunnel: w647 -> [w653] mode=indexing
          n148 = VISA Close(VISA resource name=w653) -> (error out=w655:errorcluster)  [unwired: 1 in]
          n149 = Unbundle By Name(w655) -> ("code"=→"Close Port error":i32)
        }
      }
      frame "Simulate" {
        (unwired) "This is simulation mode" ("Read")
      }
      frame "Save Setups" {
        n150 = call "!_Read-Write_Setups.vi"("Port Settings Array In"=w681, "Setup Name"="Named Serial Setup", "Mode"=enum16{"Load serial setup", "Save serial setup"}."Save serial setup") -> ()  [unwired: 2 out]
      }
    }
    n151 = Not(x="!stop") -> (.not. x?=w51:bool)
    n152 = And(x=w54, y=w51) -> (x .and. y?=w53:bool)
    "Case" <- w49
  }
  "Port Settings Array" <- w12
  "Error Description" <- w11
  "Read" <- w10
  "enumerated ports" <- w9
  "Port Initialised?" <- w8
  "Ports having file settings" <- w7
  "Audit trail" <- w5
